vi "Cal.vi"(8 "error in (no error)":errorcluster, 10 "Int Time(ms)":i32=2, 11 "Spectrum":dbl[](array[numeric])) -> (0 "error out":errorcluster, 2 "In Range?":bool, 3 "NewInt":i32)   [LabVIEW 2012]
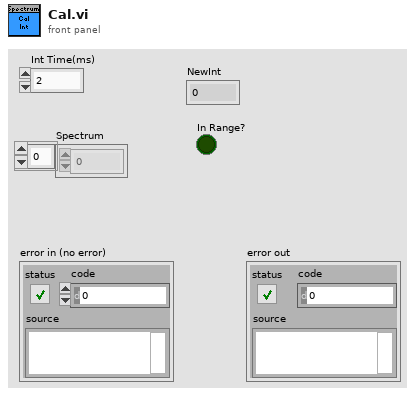
[diagram p1: front panel]
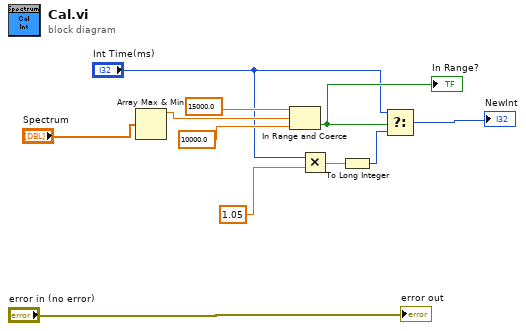
[diagram p0: block diagram]
diagram:
  n1 = Array Max & Min(array="Spectrum") -> (max value=w9:dbl)  [unwired: 3 out]
  n2 = In Range and Coerce(upper limit=15000.0, x=w9, lower limit=10000.0) -> (In Range?=w6:bool)  [unwired: 1 out]
  "In Range?" <- w6
  n3 = Multiply(x="Int Time(ms)", y=1.05) -> (x*y=w2:dbl)
  n4 = To Long Integer(number=w2) -> (32bit integer=w1:i32)
  n5 = Select(t="Int Time(ms)", s=w6, f=w1) -> (s? t:f=→"NewInt":i32)
  "error out" <- "error in (no error)"
